vi "Main Stop(FGV).vi"(1 "Method":enum16{"Get", "Put"}(ring), 3 "Stop In":bool) -> (0 "Stop Out":bool)   [LabVIEW 2015]
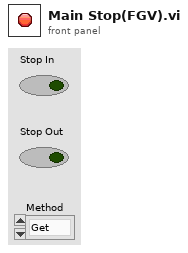
[diagram p1: front panel]
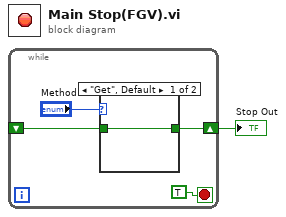
[diagram p0: block diagram]
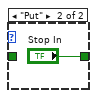
[diagram p2: hidden frame]
diagram:
  n1 = while {
    shift-right: [w4] -> w1
    shift-left: _ -> [w3]
    stop <- TRUE stop-if-true
    n2 = case shown="\"Get\", Default" "Method" {
      tunnel: [w6 "Stop In"] -> w4
      tunnel: w3 -> [w6 _]
      frame "Get", Default {
      }
      frame "Put" {
      }
    }
  }
  "Stop Out" <- w1
